vi "GenerateErrMsg.vi"(8 "error in (no error)":errorcluster, 11 "Device Model":u32) -> (0 "error out":errorcluster, 3 "Error Message":string)   [LabVIEW 2021, in "myRIOMetaDataObj.lvclass"]
uses:
  myRIOMetaDataObj.lvclass
  <vilib>/Utility/error.llb/DialogType.ctl
  InternalErrorCodes.vi
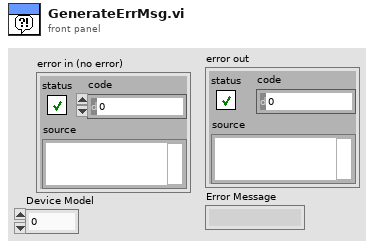
[diagram p1: front panel]
types:
  T1 = typedef "DialogType.ctl" = u16
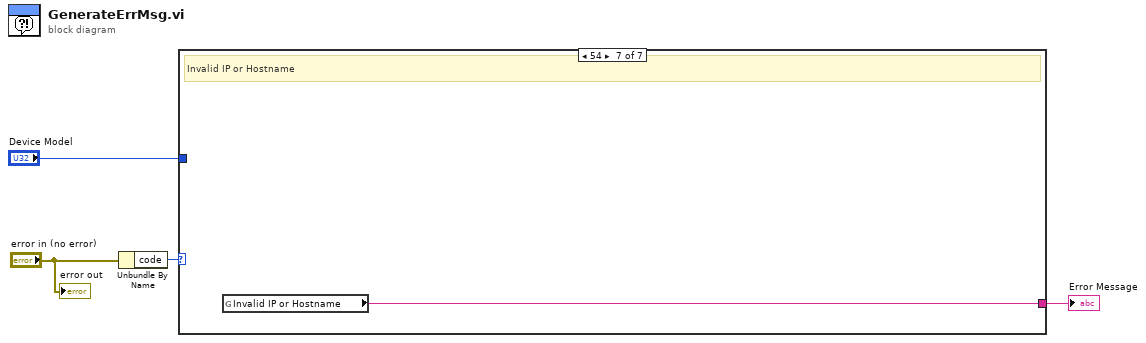
[diagram p0: block diagram]
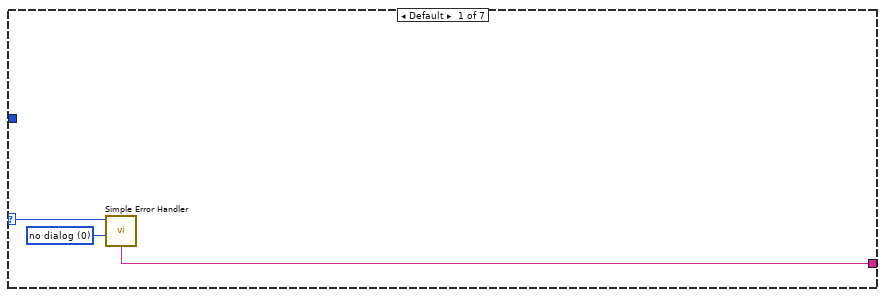
[diagram p2: hidden frame]
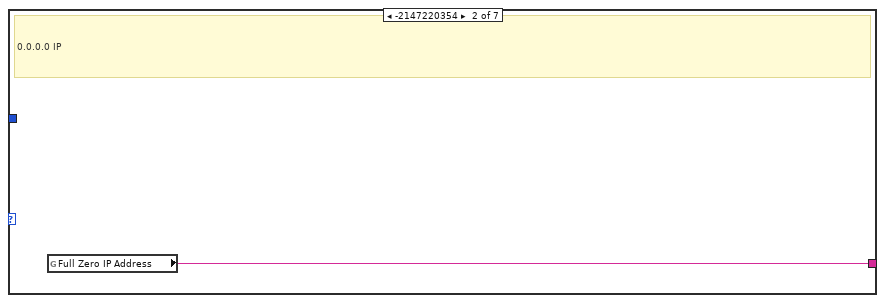
[diagram p3: hidden frame]
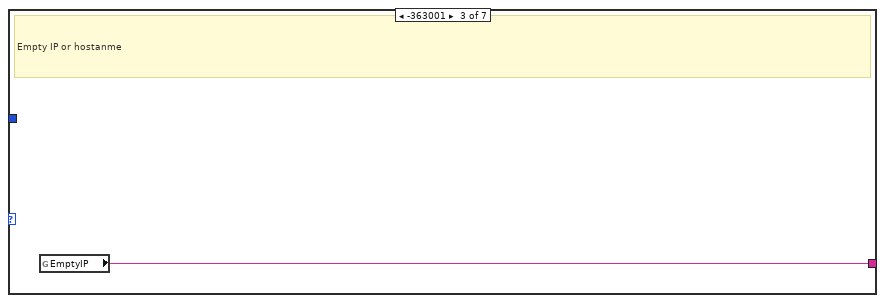
[diagram p4: hidden frame]
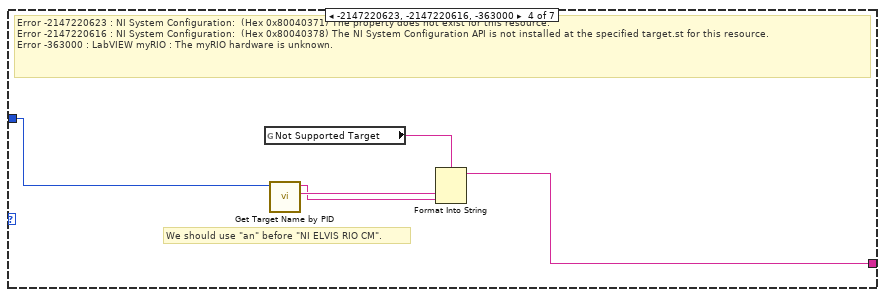
[diagram p5: hidden frame]
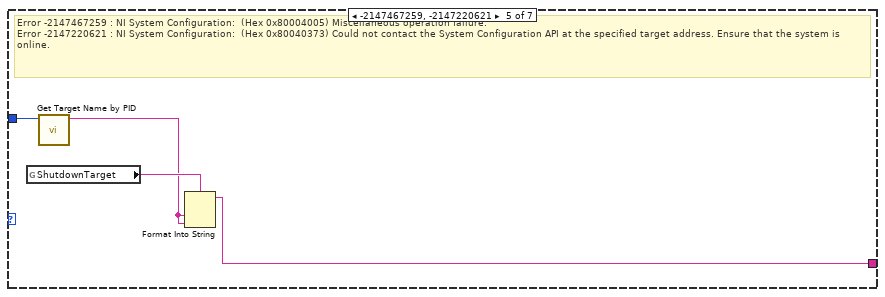
[diagram p6: hidden frame]
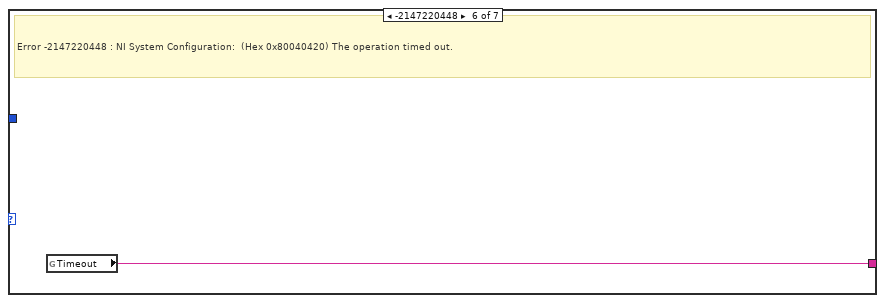
[diagram p7: hidden frame]
diagram:
  n1 = Unbundle By Name("error in (no error)") -> ("code"=w3:i32)
  n2 = case shown="54" w3 {
    selector: w3 -> [w6 _ _ _ _ _ _]
    tunnel: [w5 w8 w9 w13 w15 w19 w20] -> w2
    tunnel: "Device Model" -> [_ _ _ w14 w18 _ _]
    frame Default {
      w7 = T1 0 items=["no dialog", "OK message", "continue or stop message", "OK message + warnings", "continue/stop + warnings"] ("type of dialog (OK msg:1)")
      n3 = call <vilib>:"Simple Error Handler.vi"("error code (no error:0)"=w6, "type of dialog (OK msg:1)"=w7) -> ("message"=w5:string)  [unwired: 3 in, 4 out]
    }
    frame -2147220354 {
      # "0.0.0.0 IP"
      n4 = global read "InternalErrorCodes.vi" "Full Zero IP Address"() -> (w8:string)
    }
    frame -363001 {
      # "Empty IP or hostanme"
      n5 = global read "InternalErrorCodes.vi" "EmptyIP"() -> (w9:string)
    }
    frame -2147220623, -2147220616, -363000 {
      # "We should use \"an\" before \"NI ELVIS RIO CM\"."
      # "Error -2147220623 : NI System Configuration:  (Hex 0x80040371) The property does not exist for this resource.\nError -2147220616 : NI System Configuration:  (Hex 0x80040378) The NI System Configuration API is not installed at the specified target.st for this resource.\nError -363000 : LabVIEW myRIO : The myRIO hardware is unknown."
      n6 = global read "InternalErrorCodes.vi" "Not Supported Target"() -> (w12:string)
      n7 = call <vilib>:"Get Target Name by PID.vi"("Device Model"=w14) -> ("Article"=w11:string, "Device Model Str"=w10:string)  [unwired: 9 in]
      n8 = Format Into String(format string=w12, w11, w10) -> (resulting string=w13:string)  [unwired: 2 in, 1 out]
    }
    frame -2147467259, -2147220621 {
      # "Error -2147467259 : NI System Configuration:  (Hex 0x80004005) Miscellaneous operation failure.\nError -2147220621 : NI System Configuration:  (Hex 0x80040373) Could not contact the System Configuration API at the specified target address. Ensure that the system is online."
      n9 = global read "InternalErrorCodes.vi" "ShutdownTarget"() -> (w17:string)
      n10 = call <vilib>:"Get Target Name by PID.vi"("Device Model"=w18) -> ("Device Model Str"=w16:string)  [unwired: 9 in, 1 out]
      n11 = Format Into String(format string=w17, w16, w16) -> (resulting string=w15:string)  [unwired: 2 in, 1 out]
    }
    frame -2147220448 {
      # "Error -2147220448 : NI System Configuration:  (Hex 0x80040420) The operation timed out."
      n12 = global read "InternalErrorCodes.vi" "Timeout"() -> (w19:string)
    }
    frame 54 {
      # "Invalid IP or Hostname"
      n13 = global read "InternalErrorCodes.vi" "Invalid IP or Hostname"() -> (w20:string)
    }
  }
  "Error Message" <- w2
  "error out" <- "error in (no error)"
